vi "data_entry_string.vi"(7 "caller":refnum<vi>, 8 "error in (no error)":errorcluster, 11 "configuration":T1) -> (0 "error out":errorcluster, 2 "data_entry out":string, 3 "dialog_selection":T2)   [LabVIEW 2015, in "lv-dialog-interfaces.lvlib"]
uses:
  lv-dialog-interfaces.lvlib
  <userlib>/antonio-alexander/lv-dialog/api/v1/public/_controls/selection.ctl
  private/_controls/dialog_type.ctl
  private/_controls/hmi_references.ctl
  private/_controls/configuration.ctl
  <vilib>/event_ctls.llb/eventvkey.ctl
  <userlib>/antonio-alexander/lv-dialog/api/v1/v1.lvlib
panel:
  out "dialog":string
  in  "data_entry":string
  in  "button 1":bool
  in  "button_2":bool
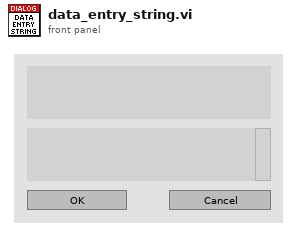
[diagram p1: front panel]
types:
  T1 = cluster{"dialog_text":string, "boolean_text_1":string, "boolean_text_2":string}
  T2 = typedef "lv-dialog.lvlib/v1.lvlib/selection.ctl" = enum16{"null", "panel_closed", "button_1", "button_2", "button_3", "cancelled"}
  T3 = typedef "lv-dialog-interfaces.lvlib/dialog_type.ctl" = enum16{"null", "one_button", "two_button", "three_button", "confirmation", "busy_wait", "error", "busy_wait_embed", "combo_box", "data_entry_string", "data_entry_numeric"}
  T4 = typedef "lv-dialog-interfaces.lvlib/configuration.ctl" = cluster{"dialog_text":string, "boolean_text_1":string, "boolean_text_2":string, "boolean_text_3":string, "inner_color":u32, "outer_color":u32, "wait_s":dbl, "error_status":bool, "error_source":string, "error_details":string, "string []":string[], "custom_entry":bool}
  T5 = typedef "lv-dialog-interfaces.lvlib/hmi_references.ctl" = cluster{"vi_reference":refnum<vi>, "caller":refnum<vi>, "dialog":refnum<vi>, "button_1":refnum<vi>, "button_2":refnum<vi>, "button_3":refnum<vi>, "busy":refnum<vi>, "error_glyph":refnum<vi>, "error_source":refnum<vi>, "error_text":refnum<vi>, "combo_box":refnum<vi>}
  T6 = typedef "eventvkey.ctl" = enum16{"ASCII", "Enter", "Return", "Shift", "Ctrl", "Alt", "Cmd", "Opt", "Caps", "NumLock", "Clear", "Break", "Up", "Down", "Left", "Right", "Insert", "Delete", "Home", "End", "PageUp", "PageDown", "Escape", "Help", "Pause", "ScrollLock", "F1", "F2", "F3", "F4", "F5", "F6", "F7", "F8", "F9", "F10", "F11", "F12", "F13", "F14", "F15", "F16", "F17", "F18", "F19", "F20", "F21", "F22", "F23", "F24", "Play", "VolumeUp", "VolumeDown", "Mute", "Two Byte Char"}
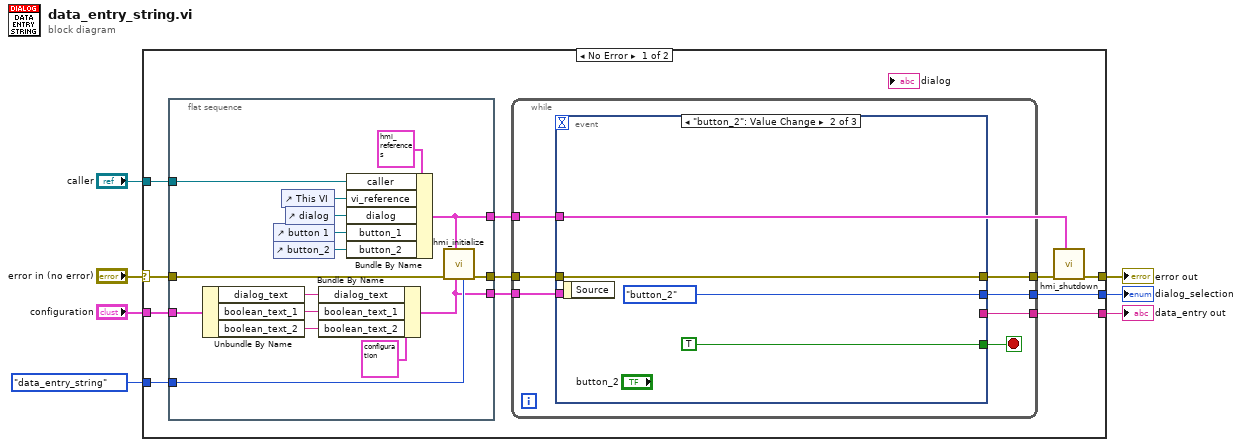
[diagram p0: block diagram]
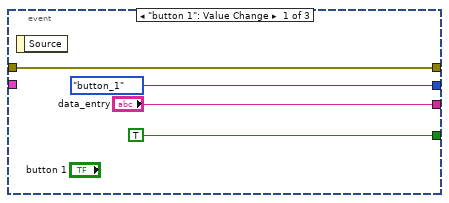
[diagram p2: hidden frame]
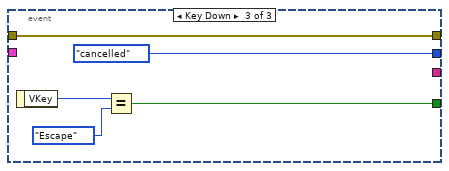
[diagram p3: hidden frame]
diagram:
  n1 = case shown="No Error" "error in (no error)" {
    selector: "error in (no error)" -> [w16 w54]
    tunnel: [w17 w54] -> w7
    tunnel: [w15 _] -> w5
    tunnel: "caller" -> [w14 _]
    tunnel: dialog_type."data_entry_string" ("dialog_type") -> [w13 _]
    tunnel: [w10 _] -> w2
    tunnel: "configuration" -> [w9 _]
    frame No Error {
      n2 = flat-sequence {
        tunnel: w16 -> [w27]
        tunnel: [w28] -> w12
        tunnel: [w23] -> w11
        tunnel: w14 -> [w32]
        tunnel: w13 -> [w26]
        tunnel: [w25] -> w8
        tunnel: w9 -> [w22]
        frame #0 {
          n3 = Unbundle By Name(w22) -> ("dialog_text"=w21:string, "boolean_text_1"=w20:string, "boolean_text_2"=w19:string)
          n4 = control-ref of="button 1"() -> (w31:refnum<vi>)
          n5 = control-ref of="button_2"() -> (w30:refnum<vi>)
          n6 = control-ref of="This VI"() -> (w33:refnum<vi>)
          n7 = control-ref of="dialog"() -> (w29:refnum<vi>)
          n8 = Bundle By Name(cluster=T4 {"dialog_text"="", "boolean_text_1"="", "boolean_text_2"="", "boolean_text_3"="", "inner_color"=16711680, "outer_color"=6618880, "wait_s"=nan, "error_status"=FALSE, "error_source"="", "error_details"="", "string []"=[], "custom_entry"=FALSE} ("configuration"), "dialog_text"=w21, "boolean_text_1"=w20, "boolean_text_2"=w19) -> (w23:T4)
          n9 = Bundle By Name(cluster=T5 {"vi_reference"=refnum, "caller"=refnum, "dialog"=refnum, "button_1"=refnum, "button_2"=refnum, "button_3"=refnum, "busy"=refnum, "error_glyph"=refnum, "error_source"=refnum, "error_text"=refnum, "combo_box"=refnum} ("references"), "caller"=w32, "vi_reference"=w33, "dialog"=w29, "button_1"=w31, "button_2"=w30) -> (w25:T5)
          n10 = call "hmi_initialize.vi"("dialog_type"=w26, "configuration"=w23, "references"=w25, "error in (no error)"=w27) -> ("error out"=w28:errorcluster)  [unwired: 7 in]
        }
      }
      n11 = while {
        tunnel: w12 -> [w38]
        tunnel: [w41] -> w15
        tunnel: w11 -> [w39]
        tunnel: [w37] -> w18
        tunnel: [w35] -> w10
        tunnel: w8 -> [w36]
        stop <- w40 stop-if-true
        n12 = event shown="[1] \"button_2\": Value Change" {
          selector: _ -> [_ _ _]
          dyn-events: _ -> [_ _ _]
          timeout: _ -> [_ _ _]
          tunnel: [selection."button_1" ("dialog_selection") selection."button_2" ("dialog_selection") selection."cancelled" ("dialog_selection")] -> w41
          tunnel: [TRUE TRUE w51] -> w40
          tunnel: w39 -> [_ _ _]
          tunnel: w38 -> [w44 w46 w52]
          tunnel: [w44 w46 w52] -> w37
          tunnel: w36 -> [_ _ _]
          tunnel: ["data_entry" _ _] -> w35
          event "button 1": Value Change {
            n13 = event-data() -> ()  [unwired: 1 in, 1 out]
          }
          event "button_2": Value Change {
            n14 = event-data() -> ()  [unwired: 1 in, 1 out]
          }
          event Key Down {
            n15 = event-data() -> ("VKey"=w50:T6)  [unwired: 1 in]
            n16 = Equal?(x=w50, y=eventvkey."Escape" ("VKey")) -> (x = y?=w51:bool)
          }
        }
      }
      n17 = call "hmi_shutdown.vi"("references"=w8, "error in (no error)"=w18) -> ("error out"=w17:errorcluster)  [unwired: 9 in]
    }
    frame Error {
    }
  }
  "error out" <- w7
  "dialog_selection" <- w5
  "data_entry out" <- w2
